vi "Set Line Interval.vi"(0 "Notifier Name":string, 7 "Line Interval":dbl, 11 "Error In":errorcluster) -> (4 "Notifier Name DUP":string, 8 "Line Interval Out":dbl, 15 "Error Out":errorcluster)   [LabVIEW 2020]
uses:
  Hardware Configuration/Hardware Configuration Controls/Company.ctl
  Hamamatsu/Orca Flash/Orca Flash Controls/Orca Flash Actions.ctl
  Hamamatsu/Orca Flash/Orca Flash Controls/Orca Flash Parameters.ctl
  Hamamatsu/Orca Flash/Orca Flash Controls/Orca Flash Parameter List.ctl
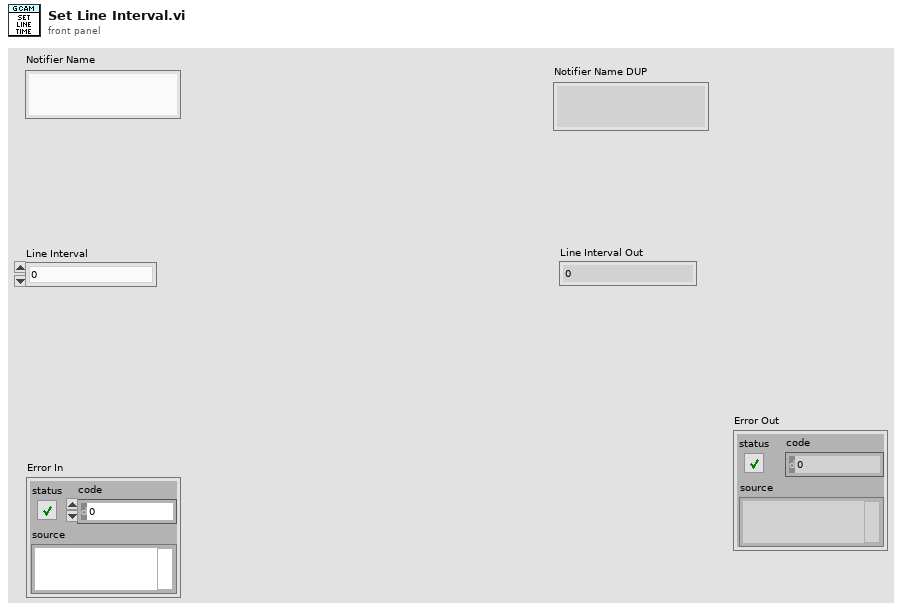
[diagram p1: front panel]
types:
  T1 = typedef "Company.ctl" = enum16{"AA Opto Electronic", "ASI", "Coherent", "Creset Optics", "CVI", "DAQmx", "Hamamatsu", "IDS", "Mad City Labs", "Marzhauser", "Measurement Computing", "MPB Com", "Photometrics", "PI", "Prior", "Thorlabs"}
  T2 = typedef "Orca Flash Parameters.ctl" = cluster{"Value":dbl, "Parameter":T3}
  T3 = typedef "Orca Flash Parameter List.ctl" = u32
  T4 = typedef "Orca Flash Actions.ctl" = enum16{"IDLE", "PREVIEW", "RECORD", "Record Settings", "SETPARAM", "GETPARAM", "SETROI", "GETROI", "PROGRESSIVE MODE", "AREA MODE", "STATUS", "QUIT"}
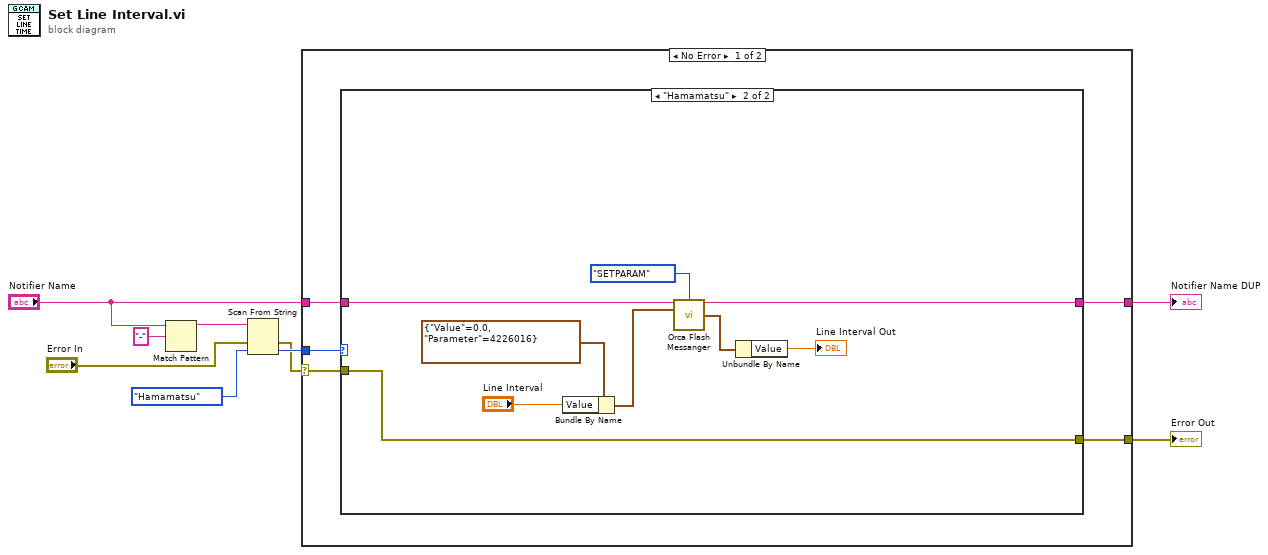
[diagram p0: block diagram]
diagram:
  n1 = Match Pattern(string="Notifier Name", regular expression="-") -> (before substring=w7:string)  [unwired: 1 in, 3 out]
  n2 = Scan From String(input string=w7, error in="Error In", default 1=Company."Hamamatsu" ("Company")) -> (error out=w3:errorcluster, output 1=w6:T1)  [unwired: 2 in, 2 out]
  n3 = case shown="No Error" w3 {
    selector: w3 -> [w12 w26]
    tunnel: w6 -> [w14 _]
    tunnel: "Notifier Name" -> [w13 w27]
    tunnel: [w11 w27] -> w2
    tunnel: [w10 w26] -> w1
    frame No Error {
      n4 = case shown="\"Hamamatsu\"" w14 {
        tunnel: w13 -> [w16 w25]
        tunnel: w12 -> [w15 w23]
        tunnel: [w16 w24] -> w11
        tunnel: [w15 w23] -> w10
        frame Default {
        }
        frame "Hamamatsu" {
          n5 = Bundle By Name(cluster=T2 {"Value"=0.0, "Parameter"=4226016} ("sCMOS Parameter"), "Value"="Line Interval") -> (w19:T2)
          n6 = call "Orca Flash Messanger.vi"("Notifier Name"=w25, "Camera Actions"=Orca_Flash_Actions."SETPARAM", "sCMOS Parameter"=w19) -> ("Notifier Name Dup"=w24:string, "sCMOS Parameter"=w18:T2)  [unwired: 8 in, 3 out]
          n7 = Unbundle By Name(w18) -> ("Value"=→"Line Interval Out":dbl)
        }
      }
    }
    frame Error {
    }
  }
  "Error Out" <- w1
  "Notifier Name DUP" <- w2
